vi "TDMS Write File.vi"(8 "error in":errorcluster, 9 "Write Settings":T2 {"Image Type" items=["Grayscale (U8)", "Grayscale (I16)", "Grayscale (SGL)", "Complex (CSG)", "RGB (U32)", "HSL (U32)", "RGB (U64)", "Grayscale (U16)"]}, 10 "Image":T3, 11 "TDMS Ref In":refnum<k34>) -> (0 "error out":errorcluster, 3 "TDMS Ref Out":refnum<k34>)   [LabVIEW 2020]
uses:
  <vilib>/vision/Image Controls.llb/IMAQ Image.ctl
  <vilib>/vision/EDVR.llb/IMAQ ImageToEDVR 1D U8.vi
  <vilib>/vision/EDVR.llb/IMAQ ImageToEDVR 1D I16.vi
  <vilib>/vision/EDVR.llb/IMAQ ImageToEDVR 1D U32.vi
  <vilib>/vision/EDVR.llb/IMAQ ImageToEDVR 1D U16.vi
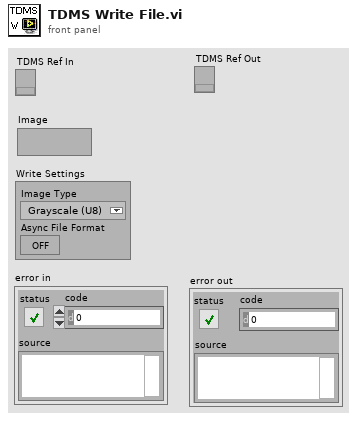
[diagram p1: front panel]
types:
  T1 = typedef "Image Type" = u32
  T2 = cluster{"Image Type":T1, "Async File Format":bool}
  T3 = typedef "IMAQ Image.ctl" = refnum<image>
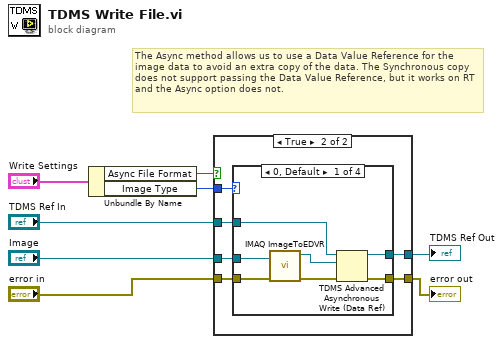
[diagram p0: block diagram]
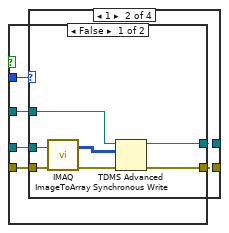
[diagram p2: hidden frame]
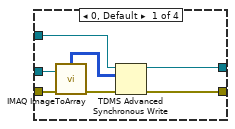
[diagram p3: hidden frame]
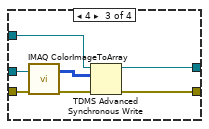
[diagram p4: hidden frame]
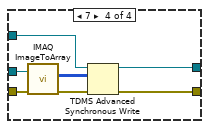
[diagram p5: hidden frame]
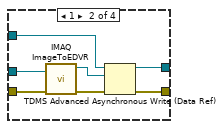
[diagram p6: hidden frame]
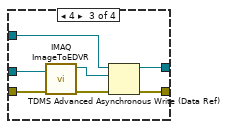
[diagram p7: hidden frame]
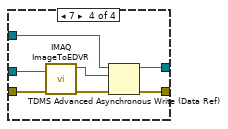
[diagram p8: hidden frame]
diagram:
  # "The Async method allows us to use a Data Value Reference for the image data to avoid an extra copy of the data. The Synchronous copy does not support passing the Data Value Reference, but it works on RT and the Async option does not."
  n1 = Unbundle By Name("Write Settings") -> ("Async File Format"=w1:bool, "Image Type"=w2:T1)
  n2 = case shown="True" w1 {
    tunnel: "Image" -> [w14 w48]
    tunnel: "TDMS Ref In" -> [w13 w46]
    tunnel: "error in" -> [w12 w47]
    tunnel: [w9 w44] -> w5
    tunnel: [w10 w43] -> w4
    tunnel: w2 -> [w11 w45]
    frame False {
      n3 = case shown="1" w11 {
        tunnel: w14 -> [w21 w28 w32 w42]
        tunnel: w12 -> [w20 w27 w31 w41]
        tunnel: w13 -> [w19 w26 w35 w40]
        tunnel: [w17 w25 w34 w39] -> w9
        tunnel: [w16 w24 w33 w38] -> w10
        frame 0, Default {
          n4 = call "IMAQ ImageToArray"("error in (no error)"=w20, "Image"=w21) -> ("error out"=w15:errorcluster, "Image Pixels (U8)"=w18:u8[][])  [unwired: 2 in, 3 out]
          n5 = TDMS Advanced Synchronous Write(8:w15, 10:w18, 11:w19) -> (0:w17:errorcluster, 3:w16:refnum<k34>)
        }
        frame 1 {
          n6 = call "IMAQ ImageToArray"("error in (no error)"=w27, "Image"=w28) -> ("error out"=w22:errorcluster, "Image Pixels (I16)"=w23:i16[][])  [unwired: 2 in, 3 out]
          n7 = TDMS Advanced Synchronous Write(8:w22, 10:w23, 11:w26) -> (0:w25:errorcluster, 3:w24:refnum<k34>)
        }
        frame 4 {
          n8 = call "IMAQ ColorImageToArray"("Image"=w32, "error in (no error)"=w31) -> ("Image Pixels (U32)"=w30:u32[][], "error out"=w29:errorcluster)  [unwired: 2 in, 1 out]
          n9 = TDMS Advanced Synchronous Write(8:w29, 10:w30, 11:w35) -> (0:w34:errorcluster, 3:w33:refnum<k34>)
        }
        frame 7 {
          n10 = call "IMAQ ImageToArray"("error in (no error)"=w41, "Image"=w42) -> ("Image Pixels (U16)"=w37:u16[][], "error out"=w36:errorcluster)  [unwired: 2 in, 3 out]
          n11 = TDMS Advanced Synchronous Write(8:w36, 10:w37, 11:w40) -> (0:w39:errorcluster, 3:w38:refnum<k34>)
        }
      }
    }
    frame True {
      n12 = case shown="0, Default" w45 {
        tunnel: w48 -> [w55 w62 w69 w76]
        tunnel: w47 -> [w54 w61 w68 w75]
        tunnel: w46 -> [w53 w60 w67 w74]
        tunnel: [w51 w58 w65 w72] -> w44
        tunnel: [w52 w59 w66 w73] -> w43
        frame 0, Default {
          n13 = call-poly <vilib>:"IMAQ ImageToEDVR.vi"("error in (no error)"=w54, "Image"=w55) -> ("error out"=w49:errorcluster, "EDVR 1D U8"=w50:refnum<data-value>)  [unwired: 7 in, 1 out]
          n14 = TDMS Advanced Asynchronous Write (Data Ref)(8:w49, 10:w50, 11:w53) -> (0:w51:errorcluster, 3:w52:refnum<k34>)  [unwired: 1 in]
        }
        frame 1 {
          n15 = call-poly <vilib>:"IMAQ ImageToEDVR.vi"("error in (no error)"=w61, "Image"=w62) -> ("error out"=w56:errorcluster, "EDVR 1D I16"=w57:refnum<data-value>)  [unwired: 7 in, 1 out]
          n16 = TDMS Advanced Asynchronous Write (Data Ref)(8:w56, 10:w57, 11:w60) -> (0:w58:errorcluster, 3:w59:refnum<k34>)  [unwired: 1 in]
        }
        frame 4 {
          n17 = call-poly <vilib>:"IMAQ ImageToEDVR.vi"("error in (no error)"=w68, "Image"=w69) -> ("error out"=w63:errorcluster, "EDVR 1D U32"=w64:refnum<data-value>)  [unwired: 7 in, 1 out]
          n18 = TDMS Advanced Asynchronous Write (Data Ref)(8:w63, 10:w64, 11:w67) -> (0:w65:errorcluster, 3:w66:refnum<k34>)  [unwired: 1 in]
        }
        frame 7 {
          n19 = call-poly <vilib>:"IMAQ ImageToEDVR.vi"("error in (no error)"=w75, "Image"=w76) -> ("error out"=w70:errorcluster, "EDVR 1D U16"=w71:refnum<data-value>)  [unwired: 7 in, 1 out]
          n20 = TDMS Advanced Asynchronous Write (Data Ref)(8:w70, 10:w71, 11:w74) -> (0:w72:errorcluster, 3:w73:refnum<k34>)  [unwired: 1 in]
        }
      }
    }
  }
  "error out" <- w5
  "TDMS Ref Out" <- w4
